vi "Evaporator Integrated Water Calculation Module (Salinity-Controled).vi"(6 "Salinity of Output Exposed\n Saline Water":dbl, 7 "Salinity of Input Exposed \nSaline Water":dbl, 8 "Lower Temp Water":dbl[unit], 9 "Higher Temp Water":dbl[unit], 10 "Mass Flow Rate of added Vapor":dbl[unit], 11 "Total Transferd Energy of Air":dbl[unit]) -> (0 "Specific Enthalpy Difference Of Pure Water":dbl[unit], 1 "Total Transfered Energy from Exposed Saline Water":dbl[unit], 2 "Mass FLow Rate of \nOutput Expose Saline Water":dbl[unit], 3 "Mass FLow Rate of \nInput Expose Saline Water":dbl[unit], 4 "S1 is greater Than S2\nThat is Wrong":bool, 5 "Mass Flow Rate of Coil Water\n& Exposed Water":dbl[unit])   [LabVIEW 2018]
panel:
  out "Mass Flow Rate of Coil Water\n& Exposed Water":dbl[unit](slide)
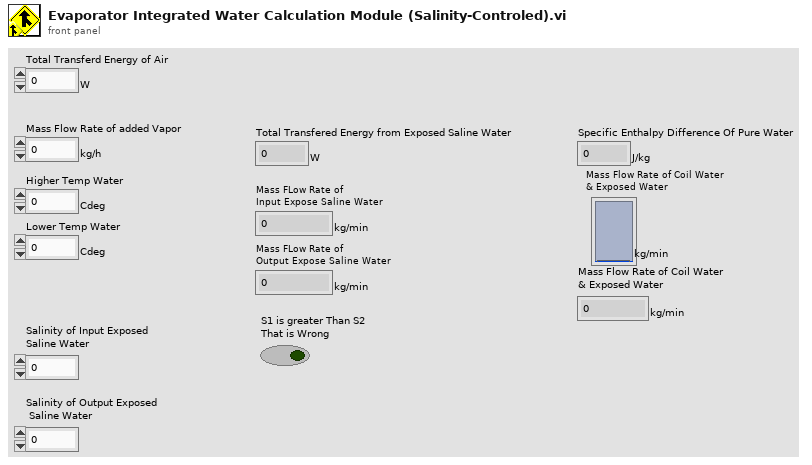
[diagram p1: front panel]
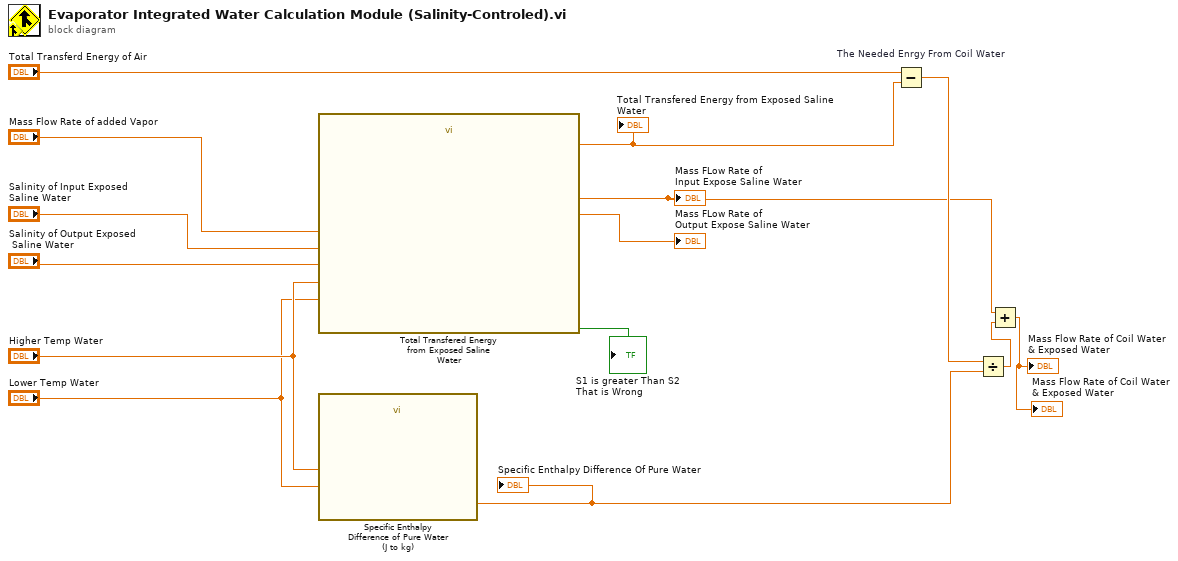
[diagram p0: block diagram]
diagram:
  n1 = call "Total Transfered Energy from Exposed Saline Water.vi"("Adde Vapor"="Mass Flow Rate of added Vapor", "Salinity Evaporator Water OUT"="Salinity of Output Exposed\n Saline Water", "Salinity Evaporator Water IN"="Salinity of Input Exposed \nSaline Water", "Lower Temp Water"="Lower Temp Water", "Higher Temp Water"="Higher Temp Water") -> ("S1 is greater Than S2\nThat is Wrong"=→"S1 is greater Than S2\nThat is Wrong":bool, "Total Transfered Energy from Exposed Saline Water"=w5:dbl[unit], "Mass FLow Rate of \nOutput Expose Saline Water"=→"Mass FLow Rate of \nOutput Expose Saline Water":dbl[unit], "Mass FLow Rate of \nInput Expose Saline Water"=w1:dbl[unit])
  "Total Transfered Energy from Exposed Saline Water" <- w5
  "Mass FLow Rate of \nInput Expose Saline Water" <- w1
  n2 = call "Specific Enthalpy Difference of Pure Water (J to kg).vi"("Lower Temp Water"="Lower Temp Water", "Higher Temp Water"="Higher Temp Water") -> ("Specific Enthalpy Difference"=w4:dbl[unit])
  "Specific Enthalpy Difference Of Pure Water" <- w4
  n3 = Subtract "The Needed Enrgy From Coil Water"(x="Total Transferd Energy of Air", y=w5) -> (x-y=w7:dbl[unit])
  n4 = Divide(x=w7, y=w4) -> (x/y=w3:dbl[unit])
  n5 = Add(x=w1, y=w3) -> (x+y=→"Mass Flow Rate of Coil Water\n& Exposed Water" →"Mass Flow Rate of Coil Water\n& Exposed Water":dbl[unit])
